vi "FeedbackDecode_PlotHeatmap.vi"(2 "Range":cluster{"Min":dbl, "Max":dbl}, 3 "InitCluster":T2={"PicPos"={"Left"=0.0, "Top"=0.0, "Width"=300.0, "Height"=300.0}, "GridSize"={"NumCol"=10.0, "NumRows"=10.0}}, 4 "GridIntensity":dbl[][](array[numeric]), 5 "MousePos":cluster{"X":i32, "Y":i32}, 6 "Instance":i32, 7 "Mode":enum16{"Initialize", "Run", "Mouse"}(ring)) -> (0 "Pic":picture, 1 "CurrPos":i32=1)   [LabVIEW 2020]
uses:
  <vilib>/imath/engines/lvmath2/RunTimeEngine/RangeToken/NIMS_Range.vi
  <instcachedir>/0/NIMS_Range_913EBD8295F041DB898D90A83F67761F.lvgen/NIMS_Range_913EBD8295F041DB898D90A83F67761F_000.vi
  <vilib>/imathl/engines/lvmath/Functions/Error Handling/Create Error.vi
  <vilib>/imath/engines/lvmath2/RunTimeSupport/NIMS_Error if Not Equal.vi
  <instcachedir>/0/NIMS_Error if Not Equal_BE0C21F4A4FB4AC7AFE883167692CC6A.lvgen/NIMS_Error if Not Equal_BE0C21F4A4FB4AC7AFE883167692CC6A_001.vi
  <vilib>/imath/engines/lvmath2/RunTimeEngine/IndexRead/NIMS V(V).vi
  <instcachedir>/0/NIMS V(V)_298D9CB7BFEB42B8BC8D9C3C28AE8C70.lvgen/NIMS V(V)_298D9CB7BFEB42B8BC8D9C3C28AE8C70_000.vi
  <vilib>/imath/engines/lvmath2/RunTimeEngine/BuiltInFunctions/meshgrid2d/NIMS_meshgrid2d(V,V).vi
  <instcachedir>/0/NIMS_meshgrid2d(V,V)_3733343E1C554A708015CFB0432C6A59.lvgen/NIMS_meshgrid2d(V,V)_3733343E1C554A708015CFB0432C6A59_000.vi
  <vilib>/imath/engines/lvmath2/RunTimeEngine/ErrorHandling/NIMS_Create Error From Enums.vi
  <vilib>/imath/engines/lvmath2/RunTimeEngine/BuiltInFunctions/reshapemx/NIMS_[GV]_reshapemx.vi
  <instcachedir>/0/NIMS_[GV]_reshapemx_116A7F60707440F78CB0D64335A3F73C.lvgen/NIMS_[GV]_reshapemx_116A7F60707440F78CB0D64335A3F73C_000.vi
  <vilib>/imath/engines/lvmath2/RunTimeEngine/RowToken/NIMS_RowToken_CV_CV.vi
  <instcachedir>/0/NIMS_RowToken_CV_CV_E2834F2F68C5494A92C49C498959A73E.lvgen/NIMS_RowToken_CV_CV_E2834F2F68C5494A92C49C498959A73E_000.vi
  <vilib>/imath/engines/lvmath2/RunTimeEngine/RowToken/NIMS_RowToken_M_CV.vi
  <instcachedir>/0/NIMS_RowToken_M_CV_79C297319A314039B767729C6880A213.lvgen/NIMS_RowToken_M_CV_79C297319A314039B767729C6880A213_000.vi
  <vilib>/imath/engines/lvmath2/RunTimeEngine/BuiltInFunctions/ones/NIMS_V=ones(I32,I32).vi
  <vilib>/imath/engines/lvmath2/RunTimeEngine/BuiltInFunctions/mod/NIMS_mod_no_size_check.vi
  <instcachedir>/0/NIMS_mod_no_size_check_5393E3382FD241D281EEB71DA286C65B.lvgen/NIMS_mod_no_size_check_5393E3382FD241D281EEB71DA286C65B_001.vi
  <vilib>/imath/engines/lvmath2/RunTimeEngine/BuiltInFunctions/length/NIMS_length(GV).vi
  <instcachedir>/0/NIMS_length(GV)_08A3D13377FD4E4B96F5795FBF3698FA.lvgen/NIMS_length(GV)_08A3D13377FD4E4B96F5795FBF3698FA_000.vi
  <instcachedir>/0/NIMS_Range_913EBD8295F041DB898D90A83F67761F.lvgen/NIMS_Range_913EBD8295F041DB898D90A83F67761F_001.vi
  <vilib>/imath/engines/lvmath2/RunTimeEngine/VariableToken/Support/NIMS_Vector Boolean Index to I32 Index.vi
  <vilib>/imath/engines/lvmath2/RunTimeEngine/IndexReplace/NIMS V(V)=M.vi
  <instcachedir>/0/NIMS V(V)=M_5A09F164FAA8499EBEBA6F6611E309D2.lvgen/NIMS V(V)=M_5A09F164FAA8499EBEBA6F6611E309D2_001.vi
  <vilib>/imath/engines/lvmath2/RunTimeEngine/BuiltInFunctions/zeros/NIMS_M=zeros(I32,I32).vi
  <vilib>/imath/engines/lvmath2/RunTimeEngine/IndexRead/NIMS V(R2).vi
  <instcachedir>/0/NIMS V(R2)_C76619605A0E4E9F8B2FA9389712AC47.lvgen/NIMS V(R2)_C76619605A0E4E9F8B2FA9389712AC47_000.vi
  <vilib>/imath/engines/lvmath2/RunTimeEngine/IndexReplace/NIMS M(V,S)=V.vi
  <instcachedir>/0/NIMS M(V,S)=V_B2FF977FD2DD4B188CCF2D61BD23E86A.lvgen/NIMS M(V,S)=V_B2FF977FD2DD4B188CCF2D61BD23E86A_000.vi
  <vilib>/imath/engines/lvmath2/RunTimeEngine/NodeEndStatement/NIMS_NodeEndStatement_Output.vi
  <instcachedir>/0/NIMS_NodeEndStatement_Output_53EC0D466D134D7ABD903AC30B43404B.lvgen/NIMS_NodeEndStatement_Output_53EC0D466D134D7ABD903AC30B43404B_001.vi
  <instcachedir>/0/NIMS_NodeEndStatement_Output_53EC0D466D134D7ABD903AC30B43404B.lvgen/NIMS_NodeEndStatement_Output_53EC0D466D134D7ABD903AC30B43404B_002.vi
  <vilib>/imath/engines/lvmath2/RunTimeEngine/ErrorHandling/NIMS_Finalize Error.vi
panel:
  out "ADim2":dbl=64.0
  in  "A":dbl[][][](array[numeric])=array5x1001x4[20020 elements]
  in  "CurrPosA":i32[](array[numeric])=[1, 1, 1, 1, 1]
  in  "PicPosA":T1(array[cluster])=[{"Left"=0.0, "Top"=50.0, "Width"=322.0, "Height"=212.0}, {"Left"=328.0, "Top"=50.0, "Width"=322.0, "Height"=212.0}, {"Left"=656.0, "Top"=50.0, "Width"=322.0, "Height"=212.0}, {"Left"=0.0, "Top"=0.0, "Width"=0.0, "Height"=0.0}, {"Left"=0.0, "Top"=0.0, "Width"=0.0, "Height"=0.0}]
  out "Jet":i32[][](array[numeric])=[[0, 0, 133], [0, 0, 143], [0, 0, 153], [0, 0, 163], [0, 0, 173], [0, 0, 184], [0, 0, 194], [0, 0, 204], [0, 0, 214], [0, 0, 224], [0, 0, 235], [0, 0, 245], [0, 0, 255], [0, 10, 255], [0, 20, 255], [0, 31, 255], [0, 41, 255], [0, 51, 255], [0, 61, 255], [0, 71, 255], [0, 82, 255], [0, 92, 255], [0, 102, 255], [0, 112, 255], [0, 122, 255], [0, 133, 255], [0, 143, 255], [0, 153, 255], [0, 163, 255], [0, 173, 255], [0, 184, 255], [0, 194, 255], [0, 204, 255], [0, 214, 255], [0, 224, 255], [0, 235, 255], [0, 245, 255], [0, 255, 255], [10, 255, 245], [20, 255, 235], [31, 255, 224], [41, 255, 214], [51, 255, 204], [61, 255, 194], [71, 255, 184], [82, 255, 173], [92, 255, 163], [102, 255, 153], [112, 255, 143], [122, 255, 133], [133, 255, 122], [143, 255, 112], [153, 255, 102], [163, 255, 92], [173, 255, 82], [184, 255, 71], [194, 255, 61], [204, 255, 51], [214, 255, 41], [224, 255, 31], [235, 255, 20], [245, 255, 10], [255, 255, 0], [255, 245, 0], [255, 235, 0], [255, 224, 0], [255, 214, 0], [255, 204, 0], [255, 194, 0], [255, 184, 0], [255, 173, 0], [255, 163, 0], [255, 153, 0], [255, 143, 0], [255, 133, 0], [255, 122, 0], [255, 112, 0], [255, 102, 0], [255, 92, 0], [255, 82, 0], [255, 71, 0], [255, 61, 0], [255, 51, 0], [255, 41, 0], [255, 31, 0], [255, 20, 0], [255, 10, 0], [255, 0, 0], [245, 0, 0], [235, 0, 0], [224, 0, 0], [214, 0, 0], [204, 0, 0], [194, 0, 0], [184, 0, 0], [173, 0, 0], [163, 0, 0], [153, 0, 0], [143, 0, 0], [133, 0, 0]]
  out "Blank":picture
  # "dim1: instance\ndim2: nR x nC\ndim3: top/left/bottom/right (length 4)"
  # "row1: channel\nrow2: intensity\nrow3: highlight"
  # "length of 2nd dim of A"
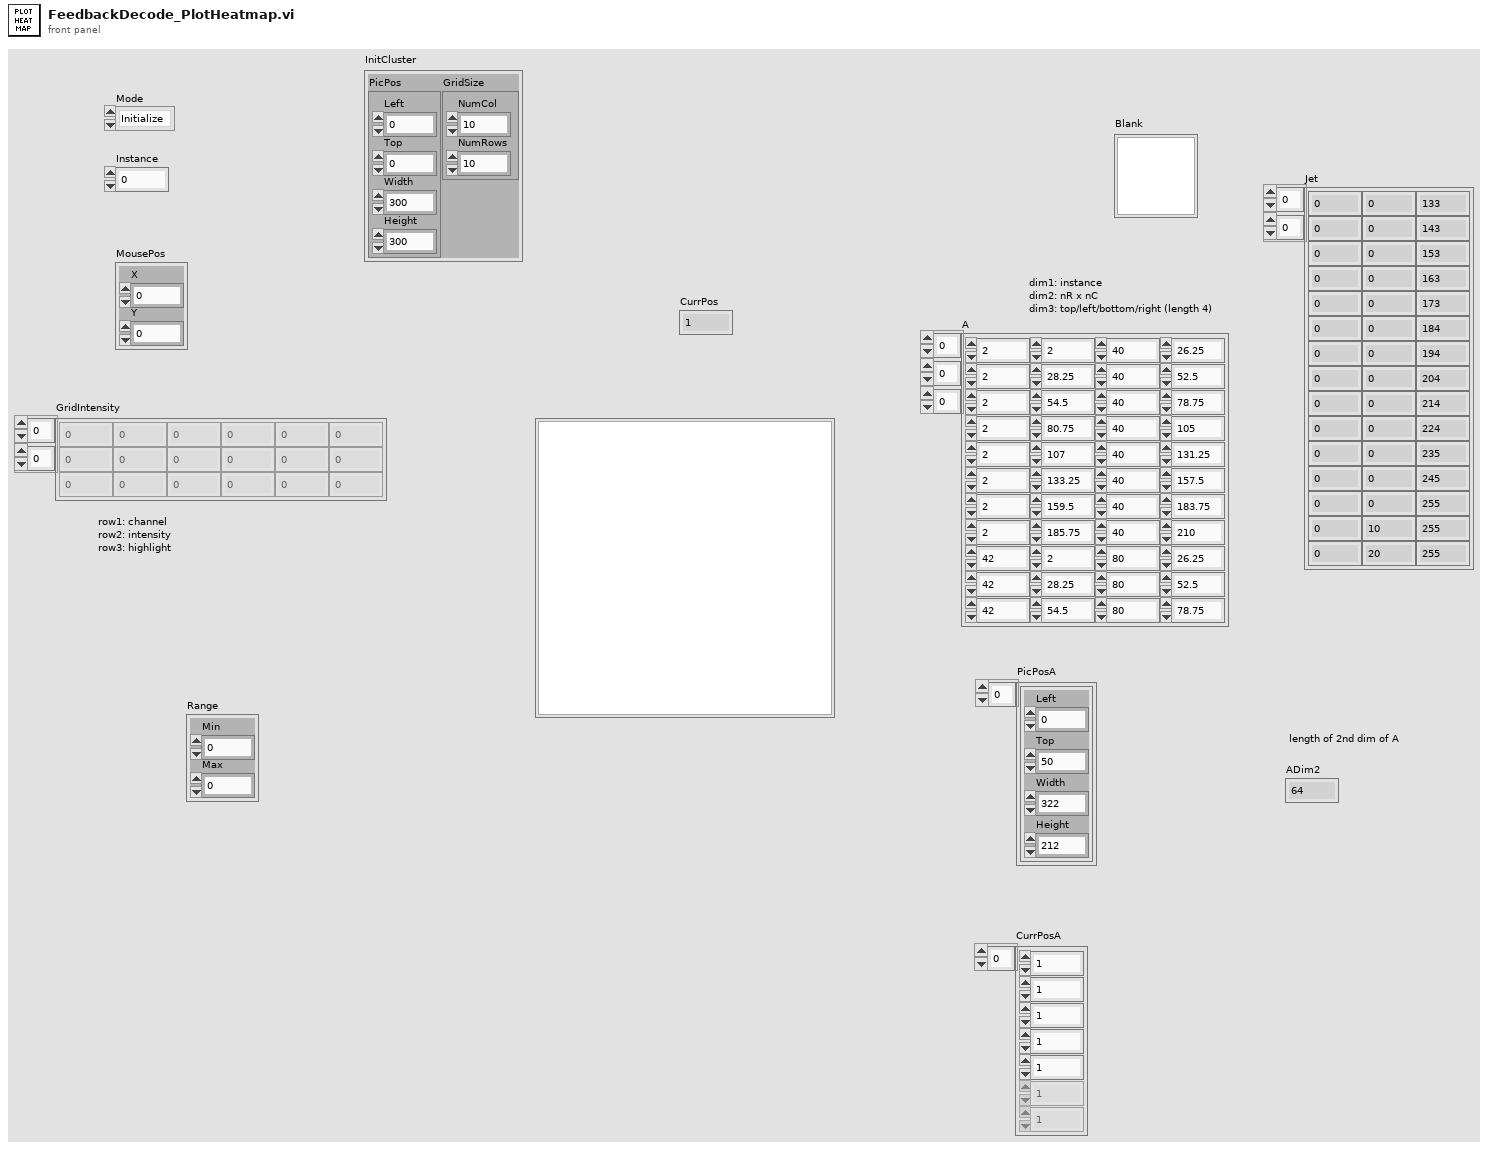
[diagram p1: front panel]
types:
  T1 = cluster{"Left":dbl, "Top":dbl, "Width":dbl, "Height":dbl}[]
  T2 = cluster{"PicPos":cluster{"Left":dbl, "Top":dbl, "Width":dbl, "Height":dbl}, "GridSize":cluster{"NumCol":dbl, "NumRows":dbl}}
  T3 = cluster{"Width":i16, "Style":enum32{"Solid", "Dash", "Dot", "DashDot", "DashDotDot"}}
  T4 = cluster{"W":dbl, "W":dbl, "Width":dbl, "Height":dbl}
  T5 = cluster{"Left":dbl, "Top":dbl, "Width":dbl, "Height":dbl}
  T6 = cluster{"[0]":dbl, "[1]":dbl, "[2]":dbl, "[3]":dbl}
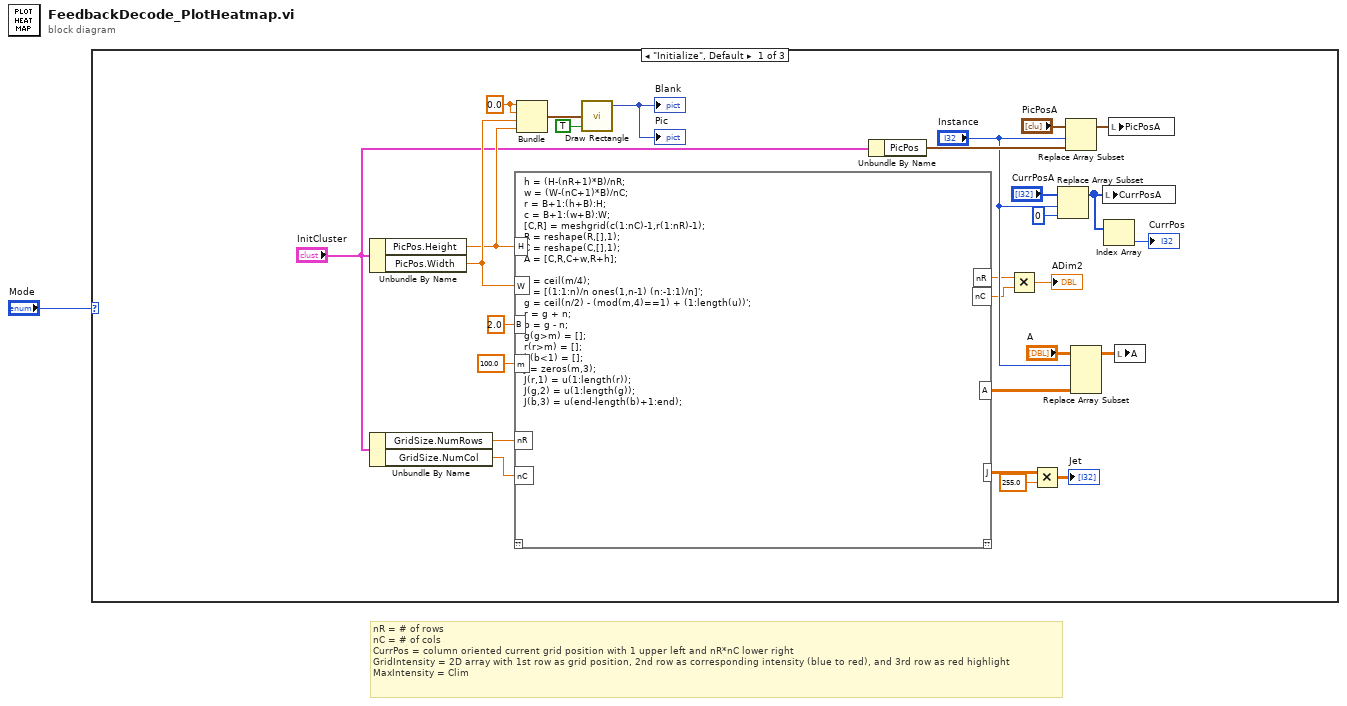
[diagram p0: block diagram]
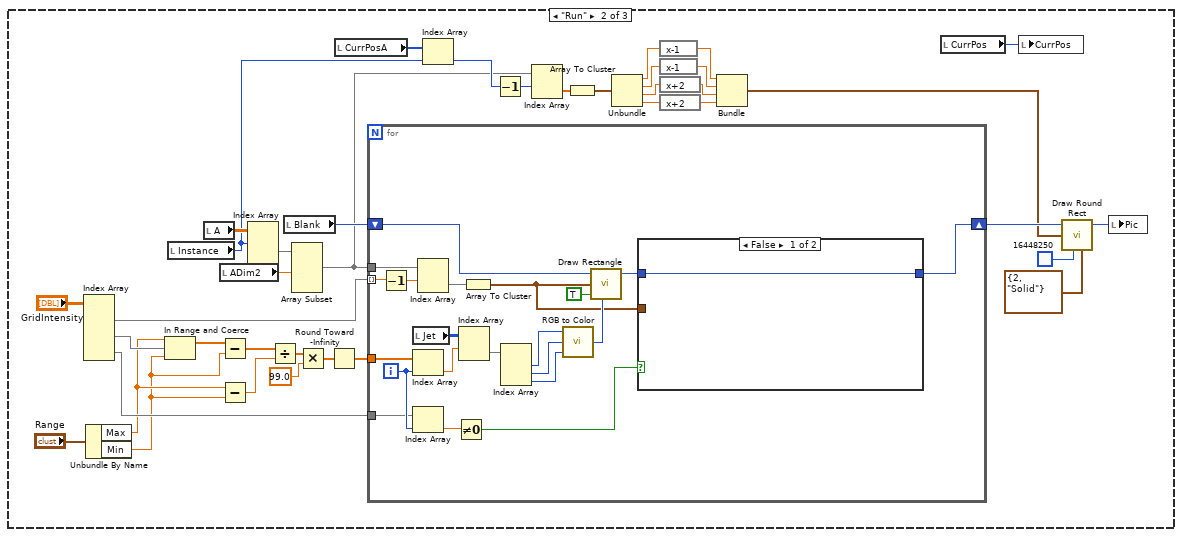
[diagram p2: hidden frame]
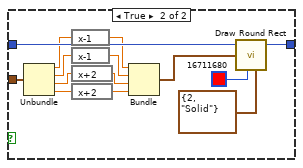
[diagram p3: hidden frame]
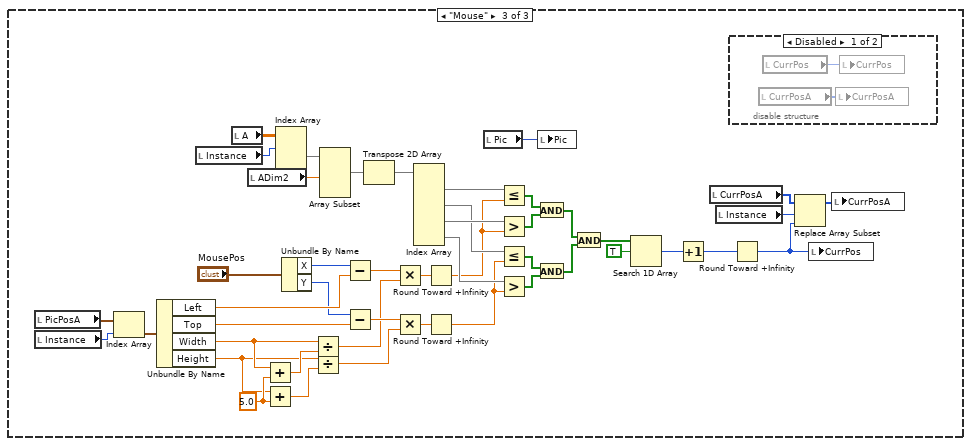
[diagram p4: hidden frame]
diagram:
  # "nR = # of rows\nnC = # of cols\nCurrPos = column oriented current grid position with 1 upper left and nR*nC lower right\nGridIntensity = 2D array with 1st row as grid position, 2nd row as corresponding intensity (blue to red), and 3rd row as red highlight\nMaxIntensity = Clim"
  n1 = case shown="\"Initialize\", Default" "Mode" {
    frame "Initialize", Default {
      w28 = 0.0 ("W")
      n2 = Unbundle By Name("InitCluster") -> ("PicPos.Height"=w18:dbl, "PicPos.Width"=w19:dbl)
      n3 = Unbundle By Name("InitCluster") -> ("GridSize.NumRows"=w21:dbl, "GridSize.NumCol"=w20:dbl)
      n4 = mathscript code="h = (H-(nR+1)*B)/nR;\nw = (W-(nC+1)*B)/nC;\nr = B+1:(h+B):H;\nc = B+1:(w+B):W;\n[C,R] = meshgrid(c(1:nC)-1,r(1:nR)-1);\nR = reshape(R,[],1);\nC = reshape(C,[],1);\nA = [C,R,C+w,R+h];\n\nn = ceil(m/4);\nu = [(1:1:n)/n ones(1,n-1) (n:-1:1)/n]';\ng = ceil(n/2) - (mod(m,4)==1) + (1:length(u))';\nr = g + n;\nb = g - n;\ng(g>m) = [];\nr(r>m) = [];\nb(b<1) = [];\nJ = zeros(m,3);\nJ(r,1) = u(1:length(r));\nJ(g,2) = u(1:length(g));\nJ(b,3) = u(end-length(b)+1:end);"("H"=w18, "W"=w19, "m"=100.0, "B"=2.0 ("m"), "nR"=w21, "nC"=w20) -> ("A"=w17:dbl[][], "J"=w25:dbl[][], "nR"=w11:dbl, "nC"=w10:dbl)  [unwired: 1 in, 1 out]
      n5 = Bundle("W"=w28, "W"=w28, "Width"=w19, "Height"=w18) -> (w27:T4)  [unwired: 1 in]
      n6 = call <vilib>:"Draw Rectangle.vi"("rect"=w27, "fill?(F)"=TRUE) -> ("new picture"=→"Blank" →"Pic":picture)  [unwired: 7 in]
      n7 = Unbundle By Name("InitCluster") -> ("PicPos"=w15:T5)
      n8 = Multiply(x=w11, y=w10) -> (x*y=→"ADim2":dbl)
      n9 = Multiply(x=w25, y=255.0) -> (x*y=→"Jet":dbl[][])
      n10 = Replace Array Subset(array="CurrPosA", new element=0 ("new element/subarray"), index="Instance") -> (w3:i32[])
      n11 = Replace Array Subset(array="PicPosA", new element=w15, index="Instance") -> (w5:T1)
      n12 = Replace Array Subset(array="A", new element=w17, index (dim 0)="Instance") -> (w8:dbl[][][])  [unwired: 2 in]
      n13 = local write "CurrPosA"(w3) -> ()
      n14 = Index Array(array=w3) -> (element=→"CurrPos":i32)  [unwired: 1 in]
      n15 = local write "PicPosA"(w5) -> ()
      n16 = local write "A"(w8) -> ()
    }
    frame "Run" {
      n17 = Index Array(array="GridIntensity") -> (element #1=w563:dbl[], element #2=w565:dbl[], element #3=w554:dbl[])  [unwired: 6 in]
      n18 = Unbundle By Name("Range") -> ("Max"=w550:dbl, "Min"=w549:dbl)
      n19 = In Range and Coerce(upper limit=w550, x=w565, lower limit=w549) -> (coerced(x)=w552:dbl[])  [unwired: 1 out]
      n20 = local read "Instance"() -> (w555:i32)
      n21 = local read "A"() -> (w559:dbl[][][])
      n22 = local read "ADim2"() -> (w557:dbl)
      n23 = Subtract(x=w552, y=w549) -> (x-y=w551:dbl[])
      n24 = Subtract(x=w550, y=w549) -> (x-y=w548:dbl)
      n25 = Index Array(array=w559, index (dim 0)=w555) -> (element=w558:dbl[][])  [unwired: 2 in]
      n26 = Divide(x=w551, y=w548) -> (x/y=w568:dbl[])
      n27 = local read "Blank"() -> (w585:picture)
      n28 = Array Subset(array=w558, length (row)=w557) -> (w556:dbl[][])  [unwired: 3 in]
      n29 = Multiply(x=w568, y=99.0) -> (x*y=w566:dbl[])
      n30 = Round Toward -Infinity(1:w566) -> (0:w564:dbl[])
      n31 = local read "CurrPosA"() -> (w562:i32[])
      n32 = for {
        tunnel: w556 -> [w596]
        tunnel: w563 -> [w606] mode=indexing
        shift-right: [w591] -> w573
        shift-left: w585 -> [w604]
        tunnel: w564 -> [w602]
        tunnel: w554 -> [w589]
        i -> [w590]
        n33 = Decrement(x=w606) -> (x-1=w595:dbl)
        n34 = local read "Jet"() -> (w601:i32[][])
        n35 = Index Array(array=w602, index=w590) -> (element=w594:dbl)
        n36 = Index Array(array=w589, index=w590) -> (element=w588:dbl)
        n37 = Index Array(array=w596, index (row)=w595) -> (element=w593:dbl[])  [unwired: 1 in]
        n38 = Not Equal To 0?(x=w588) -> (x != 0?=w587:bool)
        n39 = Index Array(array=w601, index (row)=w594) -> (element=w600:i32[])  [unwired: 1 in]
        n40 = Array To Cluster(array=w593) -> (cluster=w586:T6)
        n41 = Index Array(array=w600) -> (element #1=w599:i32, element #2=w598:i32, element #3=w597:i32)  [unwired: 3 in]
        n42 = call <vilib>:"RGB to Color.vi"("B"=w597, "G"=w598, "R"=w599) -> ("Color"=w603:u32)
        n43 = call <vilib>:"Draw Rectangle.vi"("picture"=w604, "rect"=w586, "fill?(F)"=TRUE, "color(black)"=w603) -> ("new picture"=w592:picture)  [unwired: 5 in]
        n44 = case shown="False" w587 {
          tunnel: w592 -> [w607 w619]
          tunnel: [w607 w618] -> w591
          tunnel: w586 -> [_ w609]
          frame False {
          }
          frame True {
            n45 = Unbundle(w609) -> ("[0]"=w613:dbl, "[1]"=w612:dbl, "[2]"=w611:dbl, "[3]"=w610:dbl)
            n46 = expression code="x-1"(w613) -> (w614:dbl)
            n47 = expression code="x-1"(w612) -> (w615:dbl)
            n48 = expression code="x+2"(w611) -> (w616:dbl)
            n49 = expression code="x+2"(w610) -> (w617:dbl)
            n50 = Bundle("[0]"=w614, "[1]"=w615, "[2]"=w616, "[3]"=w617) -> (w608:T6)  [unwired: 1 in]
            n51 = call <vilib>:"Draw Round Rect.vi"("picture"=w619, "rect"=w608, "color(black)"=u32 16711680, "pen"=T3 {"Width"=2, "Style"=enum."Solid"}) -> ("new picture"=w618:picture)  [unwired: 5 in]
          }
        }
      }
      n52 = Index Array(array=w562, index=w555) -> (element=w561:i32)
      n53 = Decrement(x=w561) -> (x-1=w584:i32)
      n54 = Index Array(array=w556, index (row)=w584) -> (element=w583:dbl[])  [unwired: 1 in]
      n55 = Array To Cluster(array=w583) -> (cluster=w582:T6)
      n56 = Unbundle(w582) -> ("[0]"=w578:dbl, "[1]"=w579:dbl, "[2]"=w580:dbl, "[3]"=w581:dbl)
      n57 = expression code="x-1"(w578) -> (w577:dbl)
      n58 = expression code="x-1"(w579) -> (w576:dbl)
      n59 = expression code="x+2"(w580) -> (w575:dbl)
      n60 = expression code="x+2"(w581) -> (w574:dbl)
      n61 = Bundle("[0]"=w577, "[1]"=w576, "[2]"=w575, "[3]"=w574) -> (w572:T6)  [unwired: 1 in]
      n62 = local read "CurrPos"() -> (w560:i32)
      n63 = local write "CurrPos"(w560) -> ()
      n64 = call <vilib>:"Draw Round Rect.vi"("picture"=w573, "rect"=w572, "color(black)"=u32 16448250, "pen"=T3 {"Width"=2, "Style"=enum."Solid"}) -> ("new picture"=w547:picture)  [unwired: 5 in]
      n65 = local write "Pic"(w547) -> ()
    }
    frame "Mouse" {
      w649 = 5.0 ("y")
      n66 = local read "PicPosA"() -> (w632:T1)
      n67 = local read "Instance"() -> (w633:i32)
      n68 = Index Array(array=w632, index=w633) -> (element=w631:T5)
      n69 = Unbundle By Name(w631) -> ("Left"=w651:dbl, "Top"=w652:dbl, "Width"=w648:dbl, "Height"=w646:dbl)
      n70 = local read "Instance"() -> (w627:i32)
      n71 = local read "A"() -> (w630:dbl[][][])
      n72 = local read "ADim2"() -> (w628:dbl)
      n73 = Add(x=w648, y=w649) -> (x+y=w647:dbl)
      n74 = Add(x=w646, y=w649) -> (x+y=w645:dbl)
      n75 = Index Array(array=w630, index (dim 0)=w627) -> (element=w629:dbl[][])  [unwired: 2 in]
      n76 = Unbundle By Name("MousePos") -> ("X"=w635:i32, "Y"=w634:i32)
      n77 = Divide(x=w648, y=w647) -> (x/y=w642:dbl)
      n78 = Divide(x=w646, y=w645) -> (x/y=w641:dbl)
      n79 = Array Subset(array=w629, length (row)=w628) -> (w626:dbl[][])  [unwired: 3 in]
      n80 = Subtract(x=w635, y=w651) -> (x-y=w644:dbl)
      n81 = Subtract(x=w634, y=w652) -> (x-y=w643:dbl)
      n82 = Transpose 2D Array(2D array=w626) -> (transposed array=w667:dbl[][])
      n83 = Multiply(x=w644, y=w642) -> (x*y=w640:dbl)
      n84 = Multiply(x=w643, y=w641) -> (x*y=w637:dbl)
      n85 = Index Array(array=w667) -> (element #1=w666:dbl[], element #2=w661:dbl[], element #3=w662:dbl[], element #4=w660:dbl[])  [unwired: 8 in]
      n86 = Round Toward +Infinity(x=w640) -> (ceil(x): smallest int >= x=w639:dbl)
      n87 = Round Toward +Infinity(x=w637) -> (ceil(x): smallest int >= x=w638:dbl)
      n88 = local read "Pic"() -> (w653:picture)
      n89 = Less Or Equal?(x=w666, y=w639) -> (x <= y?=w665:bool[])
      n90 = Greater?(x=w662, y=w639) -> (0:w664:bool[])
      n91 = Less Or Equal?(x=w661, y=w638) -> (x <= y?=w658:bool[])
      n92 = Greater?(x=w660, y=w638) -> (0:w659:bool[])
      n93 = And(x=w665, y=w664) -> (x .and. y?=w657:bool[])
      n94 = And(x=w658, y=w659) -> (x .and. y?=w656:bool[])
      n95 = local write "Pic"(w653) -> ()
      n96 = And(x=w657, y=w656) -> (x .and. y?=w655:bool[])
      n97 = Search 1D Array(1D array=w655, element=TRUE) -> (index of element=w654:i32)  [unwired: 1 in]
      n98 = Increment(x=w654) -> (x+1=w650:i32)
      n99 = local read "CurrPosA"() -> (w623:i32[])
      n100 = local read "Instance"() -> (w625:i32)
      n101 = disable-structure shown="Disabled" {
        frame Disabled {
          n102 = local read "CurrPosA"() -> (w669:i32[])
          n103 = local read "CurrPos"() -> (w668:i32)
          n104 = local write "CurrPosA"(w669) -> ()
          n105 = local write "CurrPos"(w668) -> ()
        }
        frame Enabled {
        }
      }
      n106 = Round Toward +Infinity(x=w650) -> (ceil(x): smallest int >= x=w622:i32)
      n107 = Replace Array Subset(array=w623, new element=w622, index=w625) -> (w624:i32[])
      n108 = local write "CurrPos"(w622) -> ()
      n109 = local write "CurrPosA"(w624) -> ()
    }
  }
